vi "Get Audio File Tags.vi"   [LabVIEW 2020, in "G-Audio.lvlib"]
doc: "<b>This VI is polymorphic.</b>\n\nRetrieve audio file tag data. Tags are returned as an array of Field \\ Value clusters, with the specified encoding applied to Value.\n\nNote that UTF-16 LE encoding is Windows only.\n\n<b>Path In</b> can be a standard path type, or a UTF-8 encoded string.\n\nSupported tag types:\nID3v2, ID3v1, Vorbis Comments, RIFF INFO"
uses:
  G-Audio.lvlib
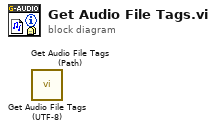
[diagram p0: block diagram]
diagram:
  n1 = call "Get Audio File Tags (UTF-8).vi"() -> ()  [unwired: 9 in, 3 out]
  n2 = call "Get Audio File Tags (Path).vi"() -> ()  [unwired: 9 in, 3 out]
